vi "MAC START.vi"(0 "System no.":i32=1 min=1 max=4 step=1, 3 "Macro name":string, 5 "error in":errorcluster, 6 "Arguments":string) -> (19 "error out":errorcluster)   [LabVIEW 2026]
doc: "Start macro. \n\nC-702, C-848, C-867, C-877, C-880, C-886, C-891, E-516, E-517, E-518, E-727, E-754, E-861 E-871, E-872, E-873, E-874: Use #8.vi to determine when macro execution has finished. For C-702, C-848, C-880, E-516 and E-517, E-518 Arguments is not supported.\n\nE-816: Use #8.vi to determine when macro execution has finished. This command cannot be issued to a slave. Check controller manual to find out if MAC START is supported. Arguments is not supported.\n\nC-887, F-206: Check HLP?/HELP answer to find out if MAC START and #8 are supported. If yes, use #8.vi to determine when macro execution has finished.\n\nC-887, M-8X0: Only for GCS syntax version = GCS 2.0 or higher (Check with CSV?.vi. If CSV?.vi is not supported, syntax version is GCS 1.0). Use #8.vi to determine when macro execution has finished.\n\nMercury: #8.vi is not supported."
panel:
  # "Start macro."
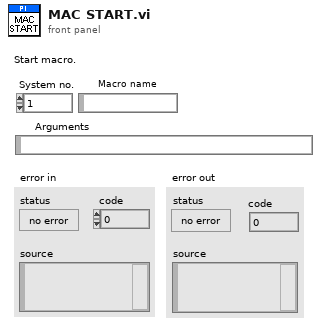
[diagram p1: front panel]
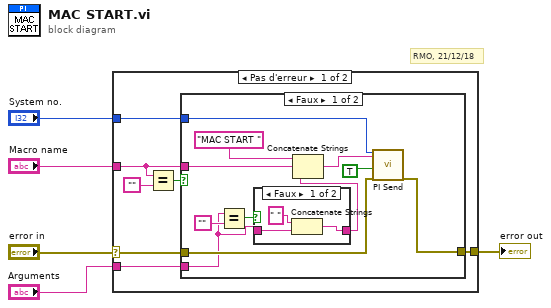
[diagram p0: block diagram]
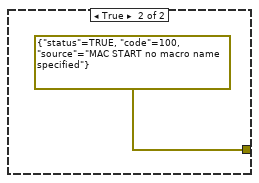
[diagram p3: hidden frame]
diagram:
  # "RMO, 21/12/18"
  n1 = case shown="Pas d'erreur" "error in" {
    selector: "error in" -> [w6 w29]
    tunnel: "System no." -> [w12 _]
    tunnel: [w11 w29] -> w4
    tunnel: "Macro name" -> [w9 _]
    tunnel: "Arguments" -> [w7 _]
    frame No Error {
      n2 = Equal?(x=w9, y="") -> (x = y?=w8:bool)
      n3 = case shown="Faux" w8 {
        tunnel: w6 -> [w23 _]
        tunnel: w12 -> [w20 _]
        tunnel: [w18 errorcluster {"status"=TRUE, "code"=100, "source"="MAC START no macro name specified"} ("error out")] -> w11
        tunnel: w9 -> [w17 _]
        tunnel: w7 -> [w14 _]
        frame False {
          n4 = Equal?(x=w14, y="") -> (x = y?=w15:bool)
          n5 = case shown="Faux" w15 {
            tunnel: w14 -> [w26 w27]
            tunnel: [w24 w27] -> w13
            frame False {
              n6 = Concatenate Strings(" ", w26) -> (w24:string)
            }
            frame True {
            }
          }
          n7 = Concatenate Strings("MAC START ", w17, w13) -> (w19:string)
          n8 = call "PI Send.vi"("System no."=w20, "String to send"=w19, "Attach termination char.?"=TRUE ("Attach Linefeed?"), "error in"=w23) -> ("error out"=w18:errorcluster)  [unwired: 2 in, 13 out]
        }
        frame True {
        }
      }
    }
    frame Error {
    }
  }
  "error out" <- w4
